vi "Sandstorm E-Stop.vi"(11 "Autonomous VI":refnum<vi>) -> (3 "Stop Sandstorm":bool)   [LabVIEW 2018]
uses:
  Robot Global Data.vi
  <vilib>/Rock Robotics/WPI/Utilities/WPI_GetSetVariantRefNum.vi
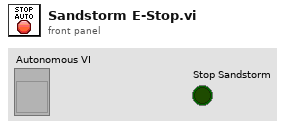
[diagram p1: front panel]
types:
  T1 = enum32{"Bad", "Idle", "Run top level", "Running"}
  T2 = typedef "WPI_JoystickDevRef.ctl" = cluster{"Device":T3}
  T3 = typedef "WPI_JoystickDeviceEnum.ctl" = enum16{"USB 0", "USB 1", "USB 2", "USB 3", "USB 4", "USB 5"}
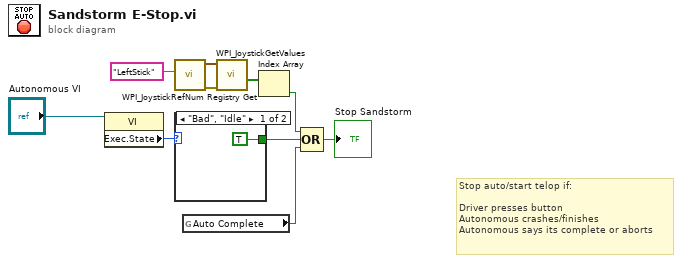
[diagram p0: block diagram]
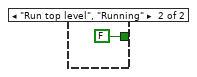
[diagram p2: hidden frame]
diagram:
  # "Stop auto/start telop if:\n\nDriver presses button\nAutonomous crashes/finishes\nAutonomous says its complete or aborts"
  n1 = property class="VI"(reference="Autonomous VI") -> ("Exec.State"=w4:T1)  [unwired: 1 in, 2 out]
  n2 = call <vilib>:"WPI_JoystickRefNum Registry Get.vi"("refnum name"="LeftStick") -> ("error out"=w9:errorcluster, "JoystickDevRef"=w8:T2)  [unwired: 9 in]
  n3 = case shown="\"Bad\", \"Idle\"" w4 {
    tunnel: [TRUE FALSE] -> w2
    frame "Bad", "Idle" {
    }
    frame "Run top level", "Running" {
    }
  }
  n4 = global read "Robot Global Data.vi" "Auto Complete"() -> (w1:bool)
  n5 = call <vilib>:"WPI_JoystickGetValues.vi"("error in (no error)"=w9, "JoystickDevRef"=w8) -> ("Buttons"=w7:bool[])  [unwired: 5 in, 4 out]
  n6 = Index Array(array=w7) -> (element=w6:bool)  [unwired: 1 in]
  n7 = Compound Arithmetic op=OR(w6, w2, w1) -> (→"Stop Sandstorm":bool)
